vi "CodeText.vi"(0 "Seq script":refnum<k24>(container)) -> ()   [LabVIEW 2019, in "XTextCode.xctl"]
uses:
  XTextCode.xctl
  System.Drawing
  System.Windows.Forms
panel:
  out "size(s)":i32
  in  "String":string="#from pulses6 import *\n#from pulses6IQindep import *\nfrom pulsesGeneric import *\n#from pulsesGenericDyn import *\n# Gate\n\ncooling = (AOM|UWAVE|MW1|MW2|MW3|MW4)\nprep = AOM|EOM\n\n\nt = True\nf = False\n\n\n\ncooltime = 6000\ndettime = 700\npreptime = 30\nrepumptime = 6\n\nprobepulse= 100\n\n#mwcheck = 6.4\nmwcheck = 120\n\ndressingpowerstep = 5\n\nclocktime1 = 715\nclocktime2 = 715\n\nmwpi = 24.4\nsbcoolcheckt = 400\nsbcoolchecktC = 1650\n\n#cpulsetime = 800\n#cpulsetime = 885\n#cpulsetime = 644\n#cpulsetime = 625\ncpulsetime = 2000\n#cpulsetime = 0\ncpulsestep = 0\n\n#sbpulsetime = 3500\n#sbpulsetime = 2000\nsbpulsetime = 2750\nsbpulsestep = 0\n\nsbfloptime = 0\nsbflopstep = 500\n\ncattime = 0\ncatstep = 300\n\ngatetime = 0\ngatestep = 300\n\ndelay = 0\nprepdelay = 500\nprepdelaystep = 0\n\n\n# Three plot experiments\n\nfindprobe             = f\nstateprep             = f\nstateprep2             = f\ndressingcheckion1     = f\ndressingcheckion2     = f\ndressingpowerscheck = f\ndressedstatescan     = f\nramseySE             = f\ndoublecat             = f\ndoublecatse         = f\ncatandgate             = f\ncatandgateparity     = f\noneloopgateSE        = f\noneloopgateparitySE    = f\ntwoloopgateSE        = f\ntwoloopgateparitySE    = f\ndetuningcheck         = f\nsidebandflop        = f\nsidebandflopC         = f\nsbcoolcheck         = f\nsbcoolcheckC         = f\ndressedstatescanAg  = f\n\n# Sideband cooling\n\nexperimentA = f\nexperiment2 = f\nexperiment3 = f\n\n\n\npulsetimespath = 'Z:\\\\iqtgroup\\\\#Projects\\\\Entanglement\\\\Pulse Sequences\\\\Sideband cooling pulse times\\\\'\n#pulsetimesfile = '200pitimes.txt'\npulsetimesfile = 'neweta50085SM467.txt'\n\n\nfile = open(pulsetimespath+pulsetimesfile)\nsbctimes = [float(line)*1e6 for line in file]\n\n\n\nstartAuxSeq()\n\n\n#expt 1 - mw probe pulse for freq stabilisation \n\n\npulse('Cooling', cooltime, 0, cooling,count = countC, AO = AO3)\npulse('AO delay', 20,0,0, AO = AO4)\npulse('Prep', preptime, 0, prep, AO = AO4)\npulse('Prep delay', prepdelay,prepdelaystep ,0)\n\nif experimentA:\n    for time in sbctimes:\n        pulse('RSB pulse', time, 0, UWAVE|XM|MW5, AO=AO4)\n        pulse('Repump', time = repumptime, dio = prep, AO = AO4)\n\n#pulse('heating delay', delay,0)\npulse('probe pulse', probepulse, 0, UWAVE|XM|MW6)\n\npulse('Detection', dettime, 0, AOM, count=countA)\npulse('Line trig set', 10,0,cooling,AO=AO3)\n\n\n\nstartMainSeq()\n\n# RF test\n\nf1=fchannel(freq=1200, amp=300, phase=0)\nf2=fchannel(freq=2200, freqstep=5, amp=350, phase=0)\nf3=fchannel(freq=1200, amp=300, phase=3.141)\nf4=fchannel(freq=4000, amp=150, phase=90)\nf5=fchannel(freq=5000, amp=100, phase=0)\nf6=fchannel(freq=6000, amp=500, phase=90)\nf7=fchannel(freq=101000, amp=300, phase=0)\nf8=fchannel(freq=101000, amp=300, phase=90)\nf9=fchannel(freq=95000, amp=100, phase=0)\nf10=fchannel(freq=100000, amp=400, phase=0)\nf11= fchannel(freq=112374.5, amp=500, phase=0*2.768)\nf12= fchannel(freq=112374.5, amp=300, phase=0*2.768)\n\nfclock1=fchannel(freq=1000, amp=600, phase=0)\nfzero=fchannel(freq=150000, amp=0, phase=0)\nfclock2=fchannel(freq=12000, amp=600, phase=0*1.57)\nfplus=fchannel(freq=10000, amp=400, phase=3.14159/2)\nfplusb=fchannel(freq=2500, amp=100, phase=3.14159/2, phasestep=0)\n\nc1 = chirpchannel(initfreq=5000, finalfreq=10000, amp=300)\nc2 = chirpchannel(initfreq=800, finalfreq=3500, amp=200)\nc3 = chirpchannel(initfreq=112324.5, finalfreq=112374.5, amp=300, ampstep = 10)\nc4 = chirpchannel(initfreq=200, finalfreq=2000, amp=300, ampstep = 0, phase = 0*3.14159)\nc5 = chirpchannel(initfreq=1024.5, finalfreq=5074.5, amp=500)\n\nm1=modchannel(amp=300, omega=2000, phi=0, b=100, nu=100, theta=0)\nm2=modchannel(amp=300, omega=1000, phi=0, b=100, nu=200, theta=0)\n\n\n## IQ mixing\n\n#rfShapedPulse('mapping pulse', time=100000, step=0, timeps=400, channels=[f1])\n#rfBlackmanPulse('mapping pulse', time=100, step=0, timeps=40, timechirp=80, channels=[c1])\n#rfBlackmanPulse('mapping pulse', time=200, step=0, timeps=40, timechirp=80, channels=[c1])\n#rfMappingPulse('mapping pulse', time=200, step=0, timeps=40, timechirp=80, channels=[c1])\n#rfMappingPulseCut('Half mapping pulse', time=200, step=0, timeps=100, timechirp=200, channels=[c1])\n#rfShapedPulse('fid measure', 10, 0, 0, [f3])\n#rfShapedPulse('fid measure', 433, 0, 20, [f1])\n#rfShapedPulse('fid measure', 0, 0, 0, [fzero])\n#rfShapedPulse('fid measure', 866, 0, 20, [f1])\n#rfShapedPulse('fid measure', 20, 0, 0, [fzero])\n#rfShapedPulse('fid measure', 433, 0, 20, [f3])\n#rfShapedPulse('fid measure', 50, 0, 0, [fzero])\n#rfShapedPulse('fid measure', 100000, 0, 50000, [f1])\n#rfShapedPulse('delay', 2000, 0, 0, [fzero])\n#rfShapedPulse('ramsey2', 10, 0, 0, [fclock2])\n#empty()\n#for n in range(20):\n#\trfShapedPulse('fid measure', 100000, 0, 50000, [f1])\n#rfMappingPulse('final pulse',time=2000, step=0, timeps=0, timechirp=1000, channels=[c3])\n#rfMappingPulse('mapping pulse',time=100, step=0, timeps=10, timechirp=0, channels=[c4])\n#rfShapedPulse('fidelity pulse',time = 30000, step=0, channels=[f12])\n#rfShapedPulse('fidelity pulse',time = 1000, step=0, channels=[f11])\n#rfMappingPulseCutEnd('Half mapping pulse', time=200, step=0, timeps=10, timechirp=200, channels=[c5])\n#rfMappingPulseCut('Half mapping pulse', time=200, step=0, timeps=10, timechirp=200, channels=[c5])\n#rfShapedPulse('fid measure', 20, 0, 0, [fplus])\n#rfShapedPulse('fid measure', 30, 0, 0, [f1])\n#rfShapedPulse('fid measure', 10, 0, 0, [fzero])\n#rfModPulse('mod pulse', 200, 0, 50, [m1,m2])\n#rfShapedPulse('pulse indep', 50, 0, 10, [fplus])\n#rfShapedPulse('pulse indep', 100, 0, 10, [fclock2])\n\n## Independent I and Q\nrfMappingPulse('mapping pulse', time=100, step=0, timeps=50, timechirp=100, IQ = 1, channels=[c4])\nrfShapedPulse('pulse indep', 50000, 0, 10, 1, [fplus])\n#rfStarkSinePulse('gate pulse', time=100, step=0, timeps=20, timechirp=5, IQ = 1, channels=[c4])\n#rfShapedPulse('pulse indep', 100, 0, 10, 1, [fclock2])\n#rfShapedPulse('pulse indep', 100000, 0, 100, 1, [fplusb])\n#for n in range(50):\n#    rfShapedPulse('pulse indep', 10000, 0, 100, 1, [fplusb])\n#rfShapedPulse('pulse indep', 100, 0, 0, 1, [fplusb])\n#rfShapedPulse('pulse indep', 200, 0, 50, 2, [fplus])\n#rfBlackmanPulse('mapping pulse', time=100, step=0, timeps=40, timechirp=80, IQ=1, channels=[c1])\n#rfModPulse('pulse indep', 100, 0, 0, 1, [m1])\n\n## Dynamic sequencing\n#rfShapedPulse('pulse indep', 100, 0, 10, 1, 1, [fplus])\n#rfBlackmanPulse('mapping pulse', time=200, step=0, timeps=40, timechirp=80, IQ=1, seg=2, channels=[c1])\n#rfMappingPulseCutEnd('mapping pulse', time=100, step=0, timeps=50, timechirp=70, IQ = 1, seg=2, channels=[c4])\n#rfModPulse('pulse indep', 100, 0, 0, 2, 1, [m1])\n#rfShapedPulse('pulse indep', 50, 0, 10, 2, 1, [fplus])\n#rfShapedPulse('pulse indep', 100, 0, 10, 1, 2, [fclock1, fplus])\n#fBlackmanPulse('mapping pulse', time=100, step=0, timeps=40, timechirp=80, IQ=2, seg=2, channels=[c1])\n\nrftime, rfstep = rfTimes()\n\n#expt 1 - mw probe pulse for freq stabilisation \n\nprobeon = f\n\npulse('Cooling', cooltime, 0, cooling,count = countC, AO = AO3)\npulse('AO delay', 20,0,0, AO = AO4)\npulse('Prep', preptime, 0, prep, AO = AO4)\npulse('Prep delay', prepdelay,prepdelaystep ,0)\n\nif (findprobe or probeon):\n    \n    pulse('probe pulse', probepulse, 0, UWAVE|XM|MW6)\n\npulse('Detection', dettime, 0, AOM, count=countA)\n\n\n\n\n\n\n#expt 2 \n\n\nion2Dcheck =         f\n\nion1dressingplus =     f\n\nion2dressingplus =     f\n\nion1clockramsey =     f\n\noffresdressing1 =     f\nion1Cscan =         f\nion1barerf =         f\n\nion1ramsey =         f\nion1ramseyse =        f\n\nion1RSBscan =         f\nion1BSBscan =         f\n\nion1cat =             f\nion1catC =             f\n\nion2cat =             f\n\nion1RSBscanC =         f\n\nion2RSBscanC =         f\n\nion2RSBscan2 =         f\n\ngateparity2 =         f\ngatese =             f\n\ntwofieldgate =         f\n\noffresrfAg =         t\n\npulse('Cooling', cooltime, 0, cooling, AO = AO3)\npulse('AO delay', 20,0,0, AO = AO4)\npulse('Prep', preptime, 0, prep, AO = AO4)\npulse('Prep delay', prepdelay,prepdelaystep ,0)\n\nif experiment2:\n    for time in sbctimes:\n        pulse('RSB pulse', time, 0, UWAVE|XM|MW5, AO=AO4)\n        pulse('Repump', time = repumptime, dio = prep, AO = AO4)\n\nif stateprep:\n    pulse('Clock pi ion 1', clocktime1, 0, UWAVE|XM|MW7)\nif stateprep2:\n    pulse('Clock pi ion 1', clocktime1, 0, UWAVE|XM|MW7)\nif sbcoolcheck:\n    pulse('RSB pulse', sbcoolcheckt , 0, UWAVE|XM|MW5)\nif sbcoolcheckC:\n    pulse('pi ion 1 +1', mwpi, 0, UWAVE|MW1)\n    pulse('RSB pulse', sbcoolchecktC, 0, UWAVE|XM|MW5)\n\nif (ion1dressingplus or findprobe or dressingcheckion1):\n    pulse('dressing ion 1 +1', mwcheck, 0, UWAVE|MW1)\n\nif dressingpowerscheck:\n    pulse('dressing powers', 0, dressingpowerstep, UWAVE|MW1|MW2|MW3|MW4)\n\nif (ion2dressingplus or dressingcheckion2):\n    pulse('dressing ion 2 +1', mwcheck, 0, UWAVE|MW3)\nif offresdressing1:\n    pulse('dressing off res 1', mwcheck,0,UWAVE|MW1|MW2|MW3|MW4)\nif ion1clockramsey:\n    pulse('clock pi ion 1', clocktime1/2, 0, UWAVE|XM|MW7)\n    pulse('delay', 0 , 500)\n    pulse('clock pi ion 1', clocktime1/2,0,UWAVE|XM|MW7)\nif (ion1Cscan or dressedstatescan):\n    pulse('clock pi ion 1', clocktime1, 0, UWAVE|XM|MW7)\n    pulse('clock pi ion 2', clocktime2, 0, UWAVE|XM|MW8)\n    pulse('ion 1 C', cpulsetime , cpulsestep , UWAVE|MW1|MW2|MW3|MW4|RF5)\n    #pulse('delay',100,0)\n    pulse('clock pi ion 1', clocktime1,0,UWAVE|XM|MW7)\n    pulse('clock pi ion 2', clocktime2, 0, UWAVE|XM|MW8)\nif dressedstatescanAg:\n    pulse('clock pi ion 1', clocktime1, 0, UWAVE|XM|MW7)\n    pulse('clock pi ion 2', clocktime2, 0, UWAVE|XM|MW8)\n    pulse('ion 1 C', cpulsetime , cpulsestep , UWAVE|MW1|MW2|MW3|MW4    |XR|AgSwitch|AgTrig)\n    pulse('clock pi ion 1', clocktime1,0,UWAVE|XM|MW7)\n    pulse('clock pi ion 2', clocktime2, 0, UWAVE|XM|MW8)\nif ion1ramsey:\n    pulse('clock pi ion 1', clocktime1, 0, UWAVE|XM|MW7)\n    pulse('clock pi ion 2', clocktime2, 0, UWAVE|XM|MW8)\n    pulse('ion 1 C', cpulsetime/2 , cpulsestep , UWAVE|MW1|MW2|MW3|MW4|RF5)\n    pulse('delay', delay, 0, UWAVE|MW1|MW2|MW3|MW4)\n    pulse('ion 1 C', cpulsetime/2 , cpulsestep , UWAVE|MW1|MW2|MW3|MW4|RF6)\n    pulse('clock pi ion 1', clocktime1,0,UWAVE|XM|MW7)\n    pulse('clock pi ion 2', clocktime2, 0, UWAVE|XM|MW8)\nif (ion1ramseyse or ramseySE):\n    pulse('clock pi ion 1', clocktime1, 0, UWAVE|XM|MW7)\n    pulse('clock pi ion 2', clocktime2, 0, UWAVE|XM|MW8)\n    pulse('ion 1 pi/2', cpulsetime/2 , cpulsestep , UWAVE|MW1|MW2|MW3|MW4|RF5)\n    pulse('delay/2', delay/2, 0, UWAVE|MW1|MW2|MW3|MW4)\n    pulse('spin echo', cpulsetime , cpulsestep , UWAVE|MW1|MW2|MW3|MW4|RF5)\n    pulse('delay/2', delay/2, 0, UWAVE|MW1|MW2|MW3|MW4)\n    pulse('ion 1 pi/2', cpulsetime/2 , cpulsestep , UWAVE|MW1|MW2|MW3|MW4|RF7)\n    pulse('clock pi ion 1', clocktime1,0,UWAVE|XM|MW7)\n    pulse('clock pi ion 2', clocktime2, 0, UWAVE|XM|MW8)\nif ion1barerf:\n    pulse('clock pi ion 1', clocktime1, 0, UWAVE|XM|MW7)\n    pulse('clock pi ion 2', clocktime2, 0, UWAVE|XM|MW8)\n    pulse('ion 1 C', cpulsetime , cpulsestep , XR|RF1|RF2|RF3|RF4)\n    pulse('clock pi ion 1', clocktime1,0,UWAVE|XM|MW7)\n    pulse('clock pi ion 2', clocktime2, 0, UWAVE|XM|MW8)\nif ion1RSBscan:\n    #pulse('heating delay', delay,0)\n    pulse('clock pi ion 1', clocktime1, 0, UWAVE|XM|MW7)\n    pulse('clock pi ion 2', clocktime2, 0, UWAVE|XM|MW8)\n    pulse('heating delay', delay,0, UWAVE|MW1|MW2|MW3|MW4)\n    pulse('ion 1 RSB', sbpulsetime , sbpulsestep , UWAVE|MW1|MW2|MW3|MW4|XR|RF1)\n    #pulse('ion 1 RSB', sbpulsetime , sbpulsestep , UWAVE|XR|RF1)\n    pulse('clock pi ion 1', clocktime1,0,UWAVE|XM|MW7)\n    pulse('clock pi ion 2', clocktime2, 0, UWAVE|XM|MW8)\nif ion1RSBscanC:\n    pulse('clock pi ion 1', clocktime1, 0, UWAVE|XM|MW7)\n    pulse('clock pi ion 2', clocktime2, 0, UWAVE|XM|MW8)\n    pulse('ion 1 C pi', cpulsetime , cpulsestep , UWAVE|MW1|MW2|MW3|MW4|RF5)\n    pulse('ion 1 RSB', sbpulsetime , sbpulsestep , UWAVE|MW1|MW2|MW3|MW4|XR|RF1)\n    pulse('ion 1 C pi', cpulsetime , cpulsestep , UWAVE|MW1|MW2|MW3|MW4|RF5)\n    #pulse('ion 1 RSB', sbpulsetime , sbpulsestep , UWAVE|XR|RF1)\n    pulse('clock pi ion 1', clocktime1,0,UWAVE|XM|MW7)\n    pulse('clock pi ion 2', clocktime2, 0, UWAVE|XM|MW8)\nif ion1BSBscan:\n    pulse('clock pi ion 1', clocktime1, 0, UWAVE|XM|MW7)\n    pulse('clock pi ion 2', clocktime2, 0, UWAVE|XM|MW8)\n    pulse('ion 1 BSB', sbpulsetime , sbpulsestep , UWAVE|MW1|MW2|MW3|MW4|XR|RF2)\n    pulse('clock pi ion 1', clocktime1,0,UWAVE|XM|MW7)\n    pulse('clock pi ion 2', clocktime2, 0, UWAVE|XM|MW8)\nif ion2RSBscan2:\n    pulse('clock pi ion 1', clocktime1, 0, UWAVE|XM|MW7)\n    pulse('clock pi ion 2', clocktime2, 0, UWAVE|XM|MW8)\n    pulse('ion 2 RSB', sbpulsetime , sbpulsestep , UWAVE|MW1|MW2|MW3|MW4|XR|RF3)\n    pulse('clock pi ion 1', clocktime1,0,UWAVE|XM|MW7)\n    pulse('clock pi ion 2', clocktime2, 0, UWAVE|XM|MW8)\nif ion2RSBscanC:\n    pulse('clock pi ion 1', clocktime1, 0, UWAVE|XM|MW7)\n    pulse('clock pi ion 2', clocktime2, 0, UWAVE|XM|MW8)\n    pulse('ion 2 C', cpulsetime , cpulsestep , UWAVE|MW1|MW2|MW3|MW4|RF6)\n    pulse('ion 2 RSB', sbpulsetime , sbpulsestep , UWAVE|MW1|MW2|MW3|MW4|XR|RF3)\n    pulse('ion 2 C', cpulsetime , cpulsestep , UWAVE|MW1|MW2|MW3|MW4|RF6)\n    pulse('clock pi ion 1', clocktime1,0,UWAVE|XM|MW7)\n    pulse('clock pi ion 2', clocktime2, 0, UWAVE|XM|MW8)\nif (ion1cat or doublecat or catandgate or catandgateparity or oneloopgateSE or oneloopgateparitySE or twoloopgateSE or twoloopgateparitySE):\n    pulse('clock pi ion 1', clocktime1, 0, UWAVE|XM|MW7)\n    pulse('clock pi ion 2', clocktime2, 0, UWAVE|XM|MW8)\n    pulse('cat ion 1', cattime , catstep , UWAVE|MW1|MW2|MW3|MW4|XR|RF1|RF2)\n    pulse('clock pi ion 1', clocktime1,0,UWAVE|XM|MW7)\n    pulse('clock pi ion 2', clocktime2, 0, UWAVE|XM|MW8)\n\nif doublecatse:\n    pulse('clock pi ion 1', clocktime1, 0, UWAVE|XM|MW7)\n    pulse('clock pi ion 2', clocktime2, 0, UWAVE|XM|MW8)\n    pulse('cat ion 1', cattime , catstep , UWAVE|MW1|MW2|MW3|MW4|XR|RF1|RF2)\n    pulse('pi', cpulsetime , cpulsestep , UWAVE|MW1|MW2|MW3|MW4|RF7|RF8)\n    pulse('delay', cattime, catstep, UWAVE|MW1|MW2|MW3|MW4)\n    pulse('clock pi ion 1', clocktime1,0,UWAVE|XM|MW7)\n    pulse('clock pi ion 2', clocktime2, 0, UWAVE|XM|MW8)\n    \n\nif ion1catC:\n    pulse('clock pi ion 1', clocktime1, 0, UWAVE|XM|MW7)\n    pulse('clock pi ion 2', clocktime2, 0, UWAVE|XM|MW8)\n    pulse('ion 1 C pi', cpulsetime , cpulsestep , UWAVE|MW1|MW2|MW3|MW4|RF5)\n    pulse('cat ion 1', cattime , catstep , UWAVE|MW1|MW2|MW3|MW4|XR|RF1|RF2)\n    pulse('ion 1 C pi', cpulsetime , cpulsestep , UWAVE|MW1|MW2|MW3|MW4|RF5)\n    pulse('clock pi ion 1', clocktime1,0,UWAVE|XM|MW7)\n    pulse('clock pi ion 2', clocktime2, 0, UWAVE|XM|MW8)\nif ion2cat:\n    pulse('clock pi ion 1', clocktime1, 0, UWAVE|XM|MW7)\n    pulse('clock pi ion 2', clocktime2, 0, UWAVE|XM|MW8)\n    pulse('cat ion 1', cattime , catstep , UWAVE|MW1|MW2|MW3|MW4|XR|RF1|RF2)\n    pulse('clock pi ion 1', clocktime1,0,UWAVE|XM|MW7)\n    pulse('clock pi ion 2', clocktime2, 0, UWAVE|XM|MW8)\nif ion2Dcheck:\n    pulse('clock pi ion 1', clocktime1, 0, UWAVE|XM|MW7)\n    pulse('clock pi ion 2', clocktime2, 0, UWAVE|XM|MW8)\n    pulse('ion 2 C', cpulsetime , cpulsestep , UWAVE|MW1|MW2|MW3|MW4|RF6)\n    pulse('clock pi ion 1', clocktime1,0,UWAVE|XM|MW7)\n    pulse('clock pi ion 2', clocktime2, 0, UWAVE|XM|MW8)\nif twofieldgate:\n    pulse('clock pi ion 1', clocktime1,0,UWAVE|XM|MW7)\n    pulse('clock pi ion 2', clocktime2, 0, UWAVE|XM|MW8)\n    pulse('gate', gatetime , gatestep , UWAVE|MW1|MW2|MW3|MW4|XR|RF2|RF3)\n    pulse('clock pi ion 1', clocktime1,0,UWAVE|XM|MW7)\n    pulse('clock pi ion 2', clocktime2,0,UWAVE|XM|MW8)\nif gateparity2:\n    pulse('clock pi ion 1', clocktime1,0,UWAVE|XM|MW7)\n    pulse('clock pi ion 2', clocktime2, 0, UWAVE|XM|MW8)\n    pulse('gate', gatetime , gatestep , UWAVE|MW1|MW2|MW3|MW4|XR|RF1|RF2|RF3|RF4)\n    pulse('both ion C', cpulsetime/2 , cpulsestep , UWAVE|MW1|MW2|MW3|MW4|RF5|RF6)\n    pulse('clock pi ion 1', clocktime1,0,UWAVE|XM|MW7)\n    pulse('clock pi ion 2', clocktime2,0,UWAVE|XM|MW8)\nif gatese:\n    pulse('clock pi ion 1', clocktime1,0,UWAVE|XM|MW7)\n    pulse('clock pi ion 2', clocktime2, 0, UWAVE|XM|MW8)\n    pulse('gate', gatetime , gatestep , UWAVE|MW1|MW2|MW3|MW4|XR|RF1|RF2|RF3|RF4)\n    pulse('pi',cpulsetime , cpulsestep , UWAVE|MW1|MW2|MW3|MW4|RF5|RF6)\n    pulse('delay',gatetime , gatestep, UWAVE|MW1|MW2|MW3|MW4)\n    pulse('clock pi ion 1', clocktime1,0,UWAVE|XM|MW7)\n    pulse('clock pi ion 2', clocktime2,0,UWAVE|XM|MW8)\nif detuningcheck:\n    pulse('clock pi ion 1', clocktime1, 0, UWAVE|XM|MW7)\n    pulse('clock pi ion 2', clocktime2, 0, UWAVE|XM|MW8)\n    pulse('ion 1 C', cpulsetime/2 , cpulsestep , UWAVE|MW1|MW2|MW3|MW4|RF5)\n    pulse('ion 1 RSB', sbpulsetime , sbpulsestep , UWAVE|MW1|MW2|MW3|MW4|XR|RF1|RF2)\n    pulse('clock pi ion 1', clocktime1,0,UWAVE|XM|MW7)\n    pulse('clock pi ion 2', clocktime2, 0, UWAVE|XM|MW8)\nif sidebandflop:\n    pulse('clock pi ion 1', clocktime1, 0, UWAVE|XM|MW7)\n    pulse('clock pi ion 2', clocktime2, 0, UWAVE|XM|MW8)\n    pulse('ion 1 RSB', sbfloptime , sbflopstep , UWAVE|MW1|MW2|MW3|MW4|XR|RF1|RF2|RF3|RF4)\n    pulse('clock pi ion 1', clocktime1,0,UWAVE|XM|MW7)\n    pulse('clock pi ion 2', clocktime2, 0, UWAVE|XM|MW8)\nif sidebandflopC:\n    pulse('clock pi ion 1', clocktime1, 0, UWAVE|XM|MW7)\n    pulse('clock pi ion 2', clocktime2, 0, UWAVE|XM|MW8)\n    pulse('ion 1 C', cpulsetime , cpulsestep , UWAVE|MW1|MW2|MW3|MW4|RF5)\n    pulse('ion 1 RSB', sbfloptime , sbflopstep , UWAVE|MW1|MW2|MW3|MW4|XR|RF1|RF2|RF3|RF4)\n    pulse('clock pi ion 1', clocktime1,0,UWAVE|XM|MW7)\n    pulse('clock pi ion 2', clocktime2, 0, UWAVE|XM|MW8)\nif offresrfAg:\n    pulse('clock pi ion 1', clocktime1,0,UWAVE|XM|MW7)\n    pulse('clock pi ion 2', clocktime2, 0, UWAVE|XM|MW8)\n    pulse('gate', gatetime , gatestep , UWAVE|XR|AgSwitch|AgTrig)\n    pulse('clock pi ion 1', clocktime1,0,UWAVE|XM|MW7)\n    pulse('clock pi ion 2', clocktime2,0,UWAVE|XM|MW8)\n\n\n\npulse('Detection', dettime, 0, AOM, count=countB)\n\n\n\n\n\n\n\n\n\n#expt 3 \n\nion1dressingminus = f\nion2dressingminus = f\n\n\nion2clockramsey =     f\n\noffresdressing2 =     f\nion2Cscan =         f\nion2barerf =         f\n\ndoubleCscan =         f\n\nion1BSBscan2 =         f\nion1BSBscan2C =     f\n\nion2RSBscan =         f\nion2BSBscan =         f\n\nion2cat =             f\nion2catC =             f\n\ngate =                 f\n\ngateC =             f\n\ntwofieldgate2 =     f\n\ngateparity =         f\ngateparityse =         f\n\ntwofieldparity =     f\n\noffresrf =             f\nsbcoolcheck2 =         f\n\npulse('Cooling', cooltime, 0, cooling, AO = AO3)\npulse('AO delay', 20,0,0, AO = AO4)\npulse('Prep', preptime, 0, prep, AO = AO4)\npulse('Prep delay', prepdelay,prepdelaystep ,0)\n\nif experiment3:\n    for time in sbctimes:\n        pulse('RSB pulse', time, 0, UWAVE|XM|MW5, AO=AO4)\n        pulse('Repump', time = repumptime, dio = prep, AO = AO4)\n\nif stateprep:\n    pulse('clock pi ion 1', clocktime1, 0, UWAVE|XM|MW7)\n    pulse('clock pi ion 2', clocktime2, 0, UWAVE|XM|MW8)\nif stateprep2:\n    pulse('clock pi ion 2', clocktime2, 0, UWAVE|XM|MW8)\nif sbcoolcheck2:\n    pulse('RSB pulse', sbcoolcheck, 0, UWAVE|XM|MW5)\nif (ion1dressingminus or dressingcheckion1):\n    pulse('dressing ion 1 -1', mwcheck, 0, UWAVE|MW2)\nif (ion2dressingminus or dressingcheckion2):\n    pulse('dressing ion 2 -1', mwcheck, 0, UWAVE|MW4)\nif offresdressing2:    \n    pulse('dressing off res 2', mwcheck,0,UWAVE|MW1|MW2|MW3|MW4)\nif ion2clockramsey:\n    pulse('clock pi ion 2', clocktime2/2, 0, UWAVE|XM|MW8)\n    pulse('delay', 0 , 500)\n    pulse('clock pi ion 2', clocktime2/2, 0, UWAVE|XM|MW8)\nif (ion2Cscan or dressedstatescan):\n    pulse('clock pi ion 1', clocktime1, 0, UWAVE|XM|MW7)\n    pulse('clock pi ion 2', clocktime2, 0, UWAVE|XM|MW8)\n    pulse('ion 2 C', cpulsetime , cpulsestep , UWAVE|MW1|MW2|MW3|MW4|RF6)\n    #pulse('delay',100,0)\n    pulse('clock pi ion 1', clocktime1,0,UWAVE|XM|MW7)\n    pulse('clock pi ion 2', clocktime2, 0, UWAVE|XM|MW8)\nif ion2barerf:\n    pulse('clock pi ion 1', clocktime1, 0, UWAVE|XM|MW7)\n    pulse('clock pi ion 2', clocktime2, 0, UWAVE|XM|MW8)\n    pulse('ion 2 C', cpulsetime , cpulsestep , XR|RF3)\n    pulse('clock pi ion 1', clocktime1,0,UWAVE|XM|MW7)\n    pulse('clock pi ion 2', clocktime2, 0, UWAVE|XM|MW8)\nif doubleCscan:\n    pulse('clock pi ion 1', clocktime1, 0, UWAVE|XM|MW7)\n    pulse('clock pi ion 2', clocktime2, 0, UWAVE|XM|MW8)\n    pulse('ion 2 C', cpulsetime , cpulsestep , UWAVE|MW1|MW2|MW3|MW4|RF5|RF6)\n    pulse('clock pi ion 1', clocktime1,0,UWAVE|XM|MW7)\n    pulse('clock pi ion 2', clocktime2, 0, UWAVE|XM|MW8)\nif ramseySE:\n    pulse('clock pi ion 1', clocktime1, 0, UWAVE|XM|MW7)\n    pulse('clock pi ion 2', clocktime2, 0, UWAVE|XM|MW8)\n    pulse('ion 1 pi/2', cpulsetime/2 , cpulsestep , UWAVE|MW1|MW2|MW3|MW4|RF6)\n    pulse('delay/2', delay/2, 0, UWAVE|MW1|MW2|MW3|MW4)\n    pulse('spin echo', cpulsetime , cpulsestep , UWAVE|MW1|MW2|MW3|MW4|RF6)\n    pulse('delay/2', delay/2, 0, UWAVE|MW1|MW2|MW3|MW4)\n    pulse('ion 1 pi/2', cpulsetime/2 , cpulsestep , UWAVE|MW1|MW2|MW3|MW4|RF8)\n    pulse('clock pi ion 1', clocktime1,0,UWAVE|XM|MW7)\n    pulse('clock pi ion 2', clocktime2, 0, UWAVE|XM|MW8)\nif ion1BSBscan2:\n    #pulse('heating delay', delay,0)\n    pulse('clock pi ion 1', clocktime1,0,UWAVE|XM|MW7)\n    pulse('clock pi ion 2', clocktime2, 0, UWAVE|XM|MW8)\n    pulse('heating delay', delay,0, UWAVE|MW1|MW2|MW3|MW4)\n    pulse('ion 1 BSB', sbpulsetime , sbpulsestep , UWAVE|MW1|MW2|MW3|MW4|XR|RF2)\n    pulse('clock pi ion 1', clocktime1,0,UWAVE|XM|MW7)\n    pulse('clock pi ion 2', clocktime2,0,UWAVE|XM|MW8)\nif ion1BSBscan2C:\n    pulse('clock pi ion 1', clocktime1,0,UWAVE|XM|MW7)\n    pulse('clock pi ion 2', clocktime2, 0, UWAVE|XM|MW8)\n    pulse('ion 2 C', cpulsetime/2 , cpulsestep , UWAVE|MW1|MW2|MW3|MW4|RF6)\n    pulse('ion 1 BSB', sbpulsetime , sbpulsestep , UWAVE|MW1|MW2|MW3|MW4|XR|RF2)\n    pulse('clock pi ion 1', clocktime1,0,UWAVE|XM|MW7)\n    pulse('clock pi ion 2', clocktime2,0,UWAVE|XM|MW8)\nif ion2RSBscan:\n    pulse('clock pi ion 1', clocktime1,0,UWAVE|XM|MW7)    \n    pulse('clock pi ion 2', clocktime2, 0, UWAVE|XM|MW8)\n    pulse('ion 2 RSB', sbpulsetime , sbpulsestep , UWAVE|MW1|MW2|MW3|MW4|XR|RF3)\n    pulse('clock pi ion 1', clocktime1,0,UWAVE|XM|MW7)\n    pulse('clock pi ion 2', clocktime2,0,UWAVE|XM|MW8)\nif ion2BSBscan:\n    pulse('clock pi ion 1', clocktime1,0,UWAVE|XM|MW7)\n    pulse('clock pi ion 2', clocktime2, 0, UWAVE|XM|MW8)\n    pulse('ion 2 BSB', sbpulsetime , sbpulsestep , UWAVE|MW1|MW2|MW3|MW4|XR|RF4)\n    pulse('clock pi ion 1', clocktime1,0,UWAVE|XM|MW7)\n    pulse('clock pi ion 2', clocktime2,0,UWAVE|XM|MW8)\nif (ion2cat or doublecat):\n    pulse('clock pi ion 1', clocktime1,0,UWAVE|XM|MW7)\n    pulse('clock pi ion 2', clocktime2, 0, UWAVE|XM|MW8)\n    pulse('ion 2 cat', cattime , catstep , UWAVE|MW1|MW2|MW3|MW4|XR|RF3|RF4)\n    pulse('clock pi ion 1', clocktime1,0,UWAVE|XM|MW7)\n    pulse('clock pi ion 2', clocktime2,0,UWAVE|XM|MW8)\nif doublecatse:\n    pulse('clock pi ion 1', clocktime1, 0, UWAVE|XM|MW7)\n    pulse('clock pi ion 2', clocktime2, 0, UWAVE|XM|MW8)\n    pulse('ion 2 cat', cattime , catstep , UWAVE|MW1|MW2|MW3|MW4|XR|RF3|RF4)\n    pulse('pi', cpulsetime , cpulsestep , UWAVE|MW1|MW2|MW3|MW4|RF7|RF8)\n    pulse('delay', cattime, catstep, UWAVE|MW1|MW2|MW3|MW4)\n    pulse('clock pi ion 1', clocktime1,0,UWAVE|XM|MW7)\n    pulse('clock pi ion 2', clocktime2, 0, UWAVE|XM|MW8)\nif ion2catC:\n    pulse('clock pi ion 1', clocktime1,0,UWAVE|XM|MW7)\n    pulse('clock pi ion 2', clocktime2, 0, UWAVE|XM|MW8)\n    pulse('ion 2 C', cpulsetime , cpulsestep , UWAVE|MW1|MW2|MW3|MW4|RF6)\n    pulse('ion 2 cat', cattime , catstep , UWAVE|MW1|MW2|MW3|MW4|XR|RF3|RF4)\n    pulse('ion 2 C', cpulsetime , cpulsestep , UWAVE|MW1|MW2|MW3|MW4|RF6)\n    pulse('clock pi ion 1', clocktime1,0,UWAVE|XM|MW7)\n    pulse('clock pi ion 2', clocktime2,0,UWAVE|XM|MW8)\nif (gate or catandgate):\n    pulse('clock pi ion 1', clocktime1,0,UWAVE|XM|MW7)\n    pulse('clock pi ion 2', clocktime2, 0, UWAVE|XM|MW8)\n    pulse('gate', gatetime , gatestep , UWAVE|MW1|MW2|MW3|MW4|XR|RF1|RF2|RF3|RF4)\n    pulse('clock pi ion 1', clocktime1,0,UWAVE|XM|MW7)\n    pulse('clock pi ion 2', clocktime2,0,UWAVE|XM|MW8)\nif gateC:\n    pulse('clock pi ion 1', clocktime1,0,UWAVE|XM|MW7)\n    pulse('clock pi ion 2', clocktime2, 0, UWAVE|XM|MW8)\n    pulse('ion 1 C', cpulsetime/2 , cpulsestep , UWAVE|MW1|MW2|MW3|MW4|RF5)\n    pulse('ion 2 C', cpulsetime/2 , cpulsestep , UWAVE|MW1|MW2|MW3|MW4|RF6)\n    pulse('gate', gatetime , gatestep , UWAVE|MW1|MW2|MW3|MW4|XR|RF1|RF2|RF3|RF4)\n    #pulse('ion 1 C', cpulsetime , cpulsestep , UWAVE|MW1|MW2|MW3|MW4|RF5)\n    #pulse('ion 2 C', cpulsetime , cpulsestep , UWAVE|MW1|MW2|MW3|MW4|RF6)\n    pulse('clock pi ion 1', clocktime1,0,UWAVE|XM|MW7)\n    pulse('clock pi ion 2', clocktime2,0,UWAVE|XM|MW8)\nif twofieldgate2:\n    pulse('clock pi ion 1', clocktime1,0,UWAVE|XM|MW7)\n    pulse('clock pi ion 2', clocktime2, 0, UWAVE|XM|MW8)\n    pulse('gate', gatetime , gatestep , UWAVE|MW1|MW2|MW3|MW4|XR|RF1|RF4)\n    pulse('clock pi ion 1', clocktime1,0,UWAVE|XM|MW7)\n    pulse('clock pi ion 2', clocktime2,0,UWAVE|XM|MW8)\nif (gateparity or catandgateparity):\n    pulse('clock pi ion 1', clocktime1,0,UWAVE|XM|MW7)\n    pulse('clock pi ion 2', clocktime2, 0, UWAVE|XM|MW8)\n    pulse('gate', gatetime , gatestep , UWAVE|MW1|MW2|MW3|MW4|XR|RF1|RF2|RF3|RF4)\n    pulse('both ion C', cpulsetime/2 , cpulsestep , UWAVE|MW1|MW2|MW3|MW4|RF5|RF6)\n    pulse('clock pi ion 1', clocktime1,0,UWAVE|XM|MW7)\n    pulse('clock pi ion 2', clocktime2,0,UWAVE|XM|MW8)\nif oneloopgateSE:\n    pulse('clock pi ion 1', clocktime1,0,UWAVE|XM|MW7)\n    pulse('clock pi ion 2', clocktime2, 0, UWAVE|XM|MW8)\n    pulse('gate', gatetime , gatestep , UWAVE|MW1|MW2|MW3|MW4|XR|RF1|RF2|RF3|RF4)\n    pulse('pi', cpulsetime , cpulsestep , UWAVE|MW1|MW2|MW3|MW4|RF7|RF8)\n    pulse('delay', gatetime, gatestep , UWAVE|MW1|MW2|MW3|MW4)\n    pulse('both ion C', cpulsetime/2 , cpulsestep , UWAVE|MW1|MW2|MW3|MW4|RF5|RF6)\n    pulse('clock pi ion 1', clocktime1,0,UWAVE|XM|MW7)\n    pulse('clock pi ion 2', clocktime2,0,UWAVE|XM|MW8)\nif oneloopgateparitySE:\n    pulse('clock pi ion 1', clocktime1,0,UWAVE|XM|MW7)\n    pulse('clock pi ion 2', clocktime2, 0, UWAVE|XM|MW8)\n    pulse('gate', gatetime , gatestep , UWAVE|MW1|MW2|MW3|MW4|XR|RF1|RF2|RF3|RF4)\n    pulse('pi', cpulsetime , cpulsestep , UWAVE|MW1|MW2|MW3|MW4|RF7|RF8)\n    pulse('delay', gatetime, gatestep , UWAVE|MW1|MW2|MW3|MW4)\n    pulse('both ion C', cpulsetime/2 , cpulsestep , UWAVE|MW1|MW2|MW3|MW4|RF5|RF6)\n    pulse('clock pi ion 1', clocktime1,0,UWAVE|XM|MW7)\n    pulse('clock pi ion 2', clocktime2,0,UWAVE|XM|MW8)\nif twoloopgateSE:\n    pulse('clock pi ion 1', clocktime1,0,UWAVE|XM|MW7)\n    pulse('clock pi ion 2', clocktime2, 0, UWAVE|XM|MW8)\n    pulse('gate 1 loop', gatetime/2 , gatestep/2 , UWAVE|MW1|MW2|MW3|MW4|XR|RF1|RF2|RF3|RF4)\n    pulse('pi', cpulsetime , cpulsestep , UWAVE|MW1|MW2|MW3|MW4|RF7|RF8)\n    pulse('gate 1 loop', gatetime/2 , gatestep/2 , UWAVE|MW1|MW2|MW3|MW4|XR|RF1|RF2|RF3|RF4)\n    pulse('clock pi ion 1', clocktime1,0,UWAVE|XM|MW7)\n    pulse('clock pi ion 2', clocktime2,0,UWAVE|XM|MW8)\nif twoloopgateparitySE:\n    pulse('clock pi ion 1', clocktime1,0,UWAVE|XM|MW7)\n    pulse('clock pi ion 2', clocktime2, 0, UWAVE|XM|MW8)\n    pulse('gate 1 loop', gatetime/2 , gatestep/2 , UWAVE|MW1|MW2|MW3|MW4|XR|RF1|RF2|RF3|RF4)\n    pulse('pi', cpulsetime , cpulsestep , UWAVE|MW1|MW2|MW3|MW4|RF7|RF8)\n    pulse('gate 1 loop', gatetime/2 , gatestep/2 , UWAVE|MW1|MW2|MW3|MW4|XR|RF1|RF2|RF3|RF4)\n    pulse('both ion C', cpulsetime/2 , cpulsestep , UWAVE|MW1|MW2|MW3|MW4|RF5|RF6)\n    pulse('clock pi ion 1', clocktime1,0,UWAVE|XM|MW7)\n    pulse('clock pi ion 2', clocktime2,0,UWAVE|XM|MW8)\nif twofieldparity:\n    pulse('clock pi ion 1', clocktime1,0,UWAVE|XM|MW7)\n    pulse('clock pi ion 2', clocktime2, 0, UWAVE|XM|MW8)\n    pulse('gate', gatetime , gatestep , UWAVE|MW1|MW2|MW3|MW4|XR|RF1|RF4)\n    pulse('ion 1 C', cpulsetime/2 , cpulsestep , UWAVE|MW1|MW2|MW3|MW4|RF5)\n    pulse('ion 2 C', cpulsetime/2 , cpulsestep , UWAVE|MW1|MW2|MW3|MW4|RF6)\n    pulse('clock pi ion 1', clocktime1,0,UWAVE|XM|MW7)\n    pulse('clock pi ion 2', clocktime2,0,UWAVE|XM|MW8)\nif offresrf:\n    pulse('clock pi ion 1', clocktime1,0,UWAVE|XM|MW7)\n    pulse('clock pi ion 2', clocktime2, 0, UWAVE|XM|MW8)\n    pulse('gate', gatetime , gatestep , UWAVE|XR|RF1|RF2|RF3|RF4)\n    pulse('clock pi ion 1', clocktime1,0,UWAVE|XM|MW7)\n    pulse('clock pi ion 2', clocktime2,0,UWAVE|XM|MW8)\n#if sidebandflop:\n    #pulse('clock pi ion 1', clocktime1, 0, UWAVE|XM|MW7)\n    #pulse('clock pi ion 2', clocktime2, 0, UWAVE|XM|MW8)\n    #pulse('ion 1 BSB', sbfloptime , sbflopstep , UWAVE|MW1|MW2|MW3|MW4|XR|RF2)\n    #pulse('clock pi ion 1', clocktime1,0,UWAVE|XM|MW7)\n    #pulse('clock pi ion 2', clocktime2, 0, UWAVE|XM|MW8)\n\n \npulse('Detection', dettime, 0, AOM, count=countD)\npulse('Line trig set', 10,0,cooling,AO=AO3)\n\n\n\n\n\n\n\n\nmakesequence()\n"
  out "TIME":u32
  out "Numeric":i32
  out "x-y":u32
  out "END":i32
  out "START":i32
  out "length":i32
  out "String 2":string
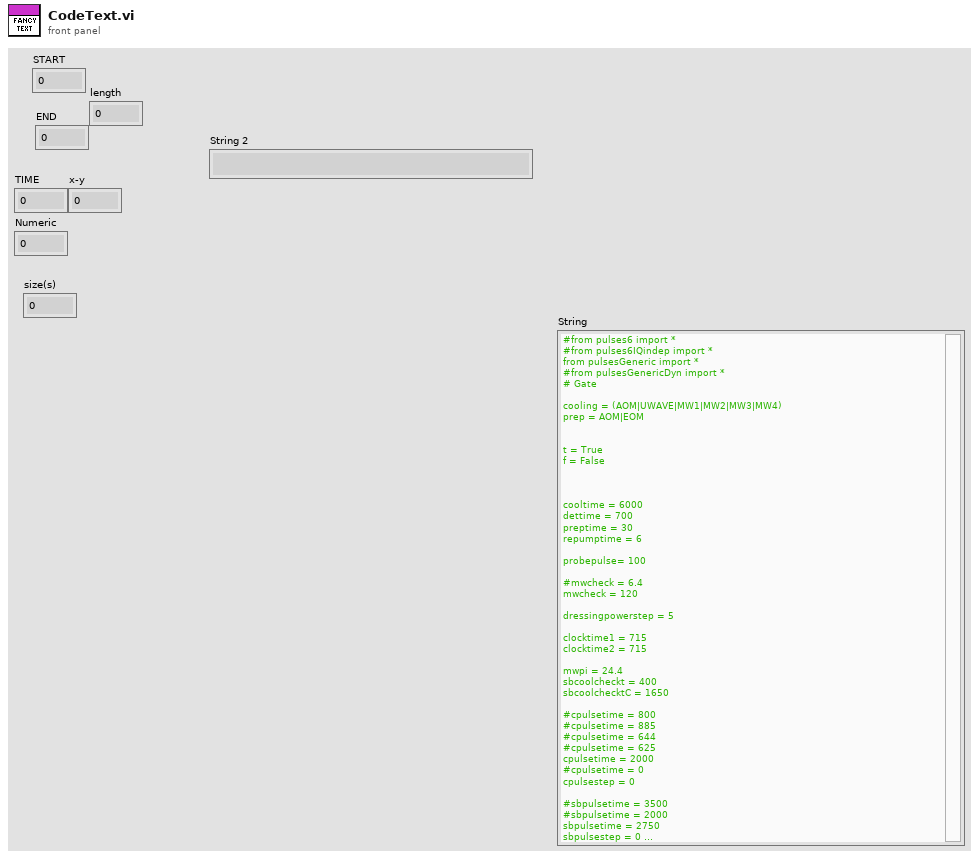
[diagram p1: front panel]
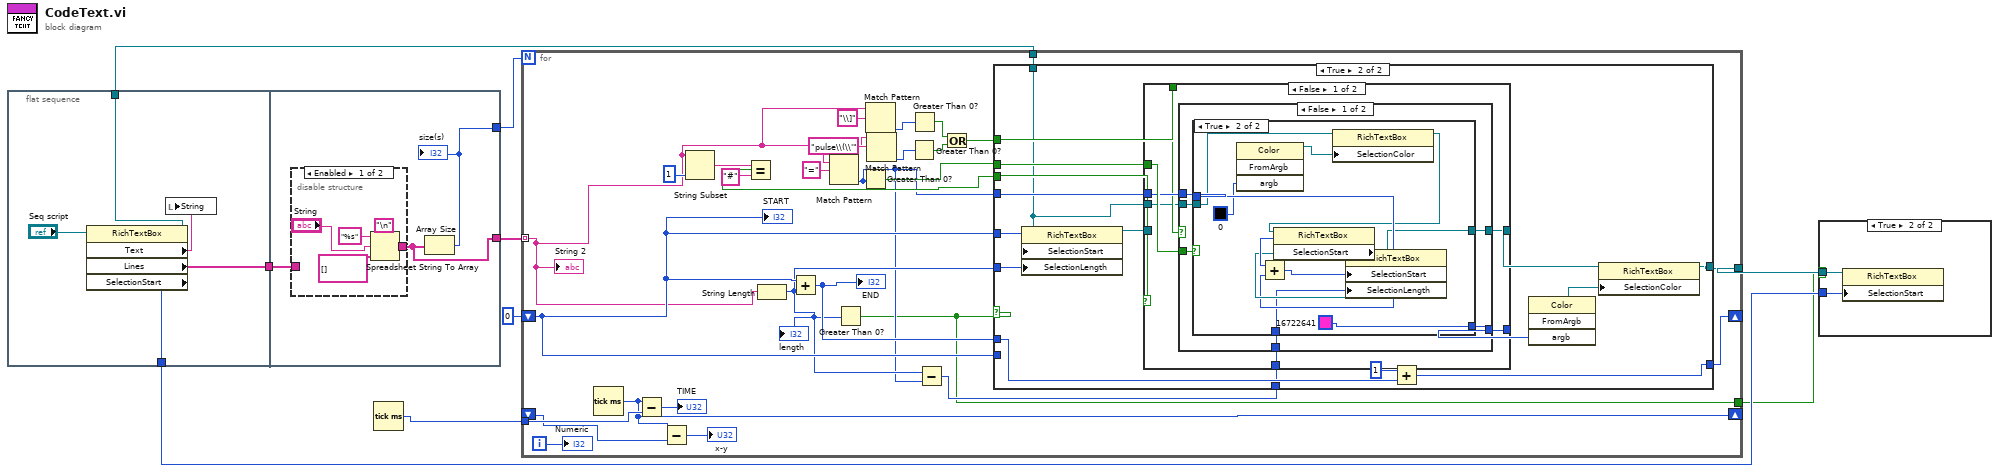
[diagram p0: block diagram]
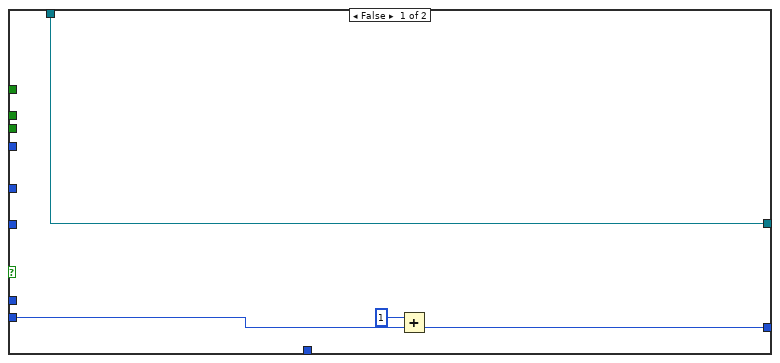
[diagram p4: hidden frame]
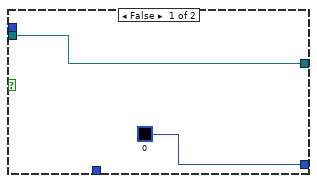
[diagram p5: hidden frame]
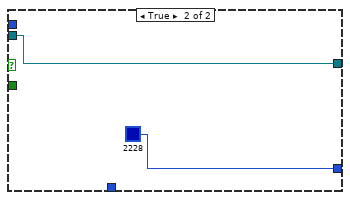
[diagram p6: hidden frame]
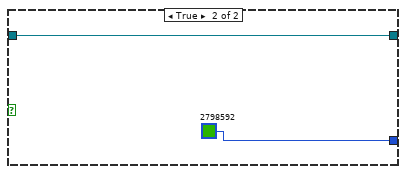
[diagram p7: hidden frame]
diagram:
  n1 = flat-sequence {
    tunnel: [w12] -> w4
    tunnel: [w13] -> w9
    tunnel: [w11] -> w2
    tunnel: [w17] -> w8
    tunnel: [w16] -> w7
    tunnel: w9 -> [w15]
    frame #0 {
      n2 = property class="RichTextBox"(reference="Seq script") -> (reference out=w12:refnum<k24>, "Text"=w14:string, "Lines"=w13:string[], "SelectionStart"=w11:i32)  [unwired: 1 in, 1 out]
      n3 = local write "String"(w14) -> ()
    }
    frame #1 {
      n4 = disable-structure shown="Enabled" {
        disable-tunnel: [w19 w23] -> w16
        disable-tunnel: w15 -> [_ w23]
        frame Enabled {
          n5 = Spreadsheet String To Array(delimiter (Tab)="\n", format string="%s", spreadsheet string="String", array type (2D Dbl)=string[] []) -> (array=w19:string[])
        }
        frame Disabled {
        }
      }
      n6 = Array Size(array=w16) -> (size(s)=w17:i32)
      "size(s)" <- w17
    }
  }
  n7 = Tick Count (ms)() -> (millisecond timer value=w6:u32)
  n8 = for {
    N: w8 -> [_]
    tunnel: w7 -> [w30] mode=indexing
    tunnel: w6 -> [w48]
    shift-right: [w44] -> _
    shift-left: _ -> [w45]
    shift-right: [w42] -> _
    shift-left: 0 -> [w41]
    tunnel: w4 -> [w35]
    tunnel: [w31] -> w3
    tunnel: [w24] -> w1
    i -> [w47]
    n9 = Tick Count (ms)() -> (millisecond timer value=w44:u32)
    n10 = Subtract(x=w44, y=w48) -> (x-y=→"TIME":u32)
    n11 = Subtract(x=w44, y=w45) -> (x-y=→"x-y":u32)
    n12 = String Subset(string=w30, length (rest)=1 ("length (rest)")) -> (substring=w50:string)  [unwired: 1 in]
    n13 = Equal?(x=w50, y="#") -> (x = y?=w37:bool)
    n14 = String Length(string=w30) -> (length=w34:i32)
    "length" <- w34
    n15 = Add(x=w41, y=w34) -> (x+y=w40:i32)
    "END" <- w40
    n16 = Match Pattern(string=w30, regular expression="=") -> (offset past match=w33:i32)  [unwired: 1 in, 3 out]
    n17 = Greater Than 0?(x=w34) -> (x > 0?=w24:bool)
    n18 = Greater Than 0?(x=w33) -> (x > 0?=w36:bool)
    n19 = Match Pattern(string=w30, regular expression="\\]") -> (offset past match=w28:i32)  [unwired: 1 in, 3 out]
    n20 = Match Pattern(string=w30, regular expression="pulse\\(\\'") -> (offset past match=w38:i32)  [unwired: 1 in, 3 out]
    n21 = Greater Than 0?(x=w38) -> (x > 0?=w27:bool)
    n22 = Greater Than 0?(x=w28) -> (x > 0?=w26:bool)
    n23 = Subtract(x=w34, y=w33) -> (x-y=w32:i32)
    n24 = Or(x=w26, y=w27) -> (x .or. y?=w25:bool)
    n25 = case shown="True" w24 {
      tunnel: w37 -> [_ w72]
      tunnel: w36 -> [_ w71]
      tunnel: w33 -> [_ w70]
      tunnel: w40 -> [_ w69]
      tunnel: [w55 w68] -> w42
      tunnel: w41 -> [w56 _]
      tunnel: w41 -> [_ w67]
      tunnel: w34 -> [_ w66]
      tunnel: w25 -> [_ w65]
      tunnel: w35 -> [w53 w64]
      tunnel: w32 -> [_ w60]
      tunnel: [w53 w57] -> w31
      frame False {
        n26 = Add(x=1, y=w56) -> (x+y=w55:i32)
      }
      frame True {
        n27 = property on="Property Node" class="RichTextBox"(reference=w64, "SelectionStart"=w67, "SelectionLength"=w66) -> (reference out=w59:refnum<k24>)  [unwired: 1 in, 1 out]
        n28 = case shown="False" w72 {
          tunnel: [w79 u32 2798592 ("Color Box 2")] -> w62
          tunnel: w71 -> [w78 _]
          tunnel: w70 -> [w77 _]
          tunnel: w65 -> [w76 _]
          tunnel: w64 -> [w75 _]
          tunnel: w60 -> [w74 _]
          tunnel: w59 -> [_ w102]
          tunnel: [w73 w102] -> w58
          frame False {
            n29 = case shown="False" w76 {
              tunnel: [w85 u32 2228 ("Color Box 2")] -> w79
              tunnel: w78 -> [w84 _]
              tunnel: w77 -> [w83 _]
              tunnel: w75 -> [w82 w100]
              tunnel: w74 -> [w81 _]
              tunnel: [w80 w100] -> w73
              frame False {
                n30 = case shown="True" w84 {
                  tunnel: [u32 0 ("Color Box 2") u32 16722641 ("Color Box 2")] -> w85
                  tunnel: w83 -> [_ w94]
                  tunnel: w82 -> [w86 w91]
                  tunnel: w81 -> [_ w93]
                  tunnel: [w86 w92] -> w80
                  frame False {
                  }
                  frame True {
                    n31 = invoke class="Color" method="FromArgb"("argb"=u32 0 ("Color Box 2")) -> (reference out=w89:refnum<k24>)  [unwired: 3 in, 3 out]
                    n32 = property on="Property Node" class="RichTextBox"(reference=w91, "SelectionColor"=w89) -> (reference out=w90:refnum<k24>)  [unwired: 1 in, 1 out]
                    n33 = property on="Property Node" class="RichTextBox"(reference=w90) -> (reference out=w95:refnum<k24>, error out=w96:errorcluster, "SelectionStart"=w98:i32)  [unwired: 1 in]
                    n34 = Add(x=w98, y=w94) -> (x+y=w99:i32)
                    n35 = property on="Property Node" class="RichTextBox"(reference=w95, error in=w96, "SelectionStart"=w99, "SelectionLength"=w93) -> (reference out=w92:refnum<k24>)  [unwired: 1 out]
                  }
                }
              }
              frame True {
              }
            }
          }
          frame True {
          }
        }
        n36 = Add(x=1, y=w69) -> (x+y=w68:i32)
        n37 = invoke class="Color" method="FromArgb"("argb"=w62) -> ("FromArgb"=w63:refnum<k24>)  [unwired: 3 in, 3 out]
        n38 = property on="Property Node" class="RichTextBox"(reference=w58, "SelectionColor"=w63) -> (reference out=w57:refnum<k24>)  [unwired: 1 in, 1 out]
      }
    }
    "Numeric" <- w47
    "START" <- w41
    "String 2" <- w30
  }
  n39 = case shown="True" w1 {
    tunnel: w3 -> [_ w105]
    tunnel: w2 -> [_ w104]
    frame False {
    }
    frame True {
      n40 = property class="RichTextBox"(reference=w105, "SelectionStart"=w104) -> ()  [unwired: 1 in, 2 out]
    }
  }
